vi "insert into cost so far.vi"(9 "new cost":dbl, 10 "Node":cluster{"Weight":dbl, "Row":dbl, "Col":dbl}, 11 "Cost_so_far":T1(array[cluster])) -> (3 "cost_so_far output":T1(array[cluster]))   [LabVIEW 2014]
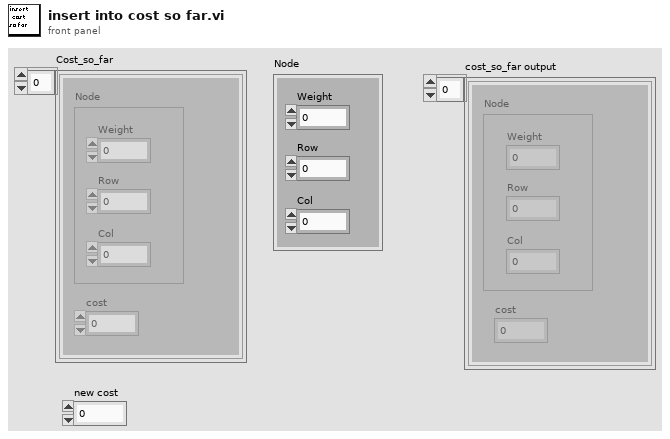
[diagram p1: front panel]
types:
  T1 = cluster{"Node":cluster{"Weight":dbl, "Row":dbl, "Col":dbl}, "cost":dbl}[]
  T2 = cluster{"Node":cluster{"Weight":dbl, "Row":dbl, "Col":dbl}, "cost":dbl}
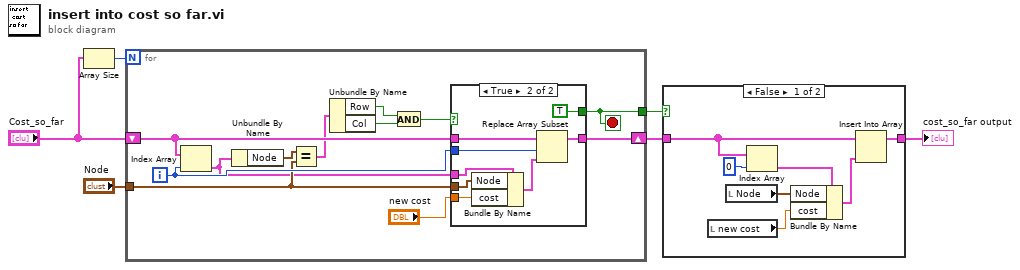
[diagram p0: block diagram]
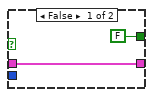
[diagram p3: hidden frame]
diagram:
  n1 = Array Size(array="Cost_so_far") -> (size(s)=w6:i32)
  n2 = for {
    N: w6 -> [_]
    tunnel: "Node" -> [w15]
    shift-right: [w12] -> w2
    shift-left: "Cost_so_far" -> [w17]
    tunnel: [w11] -> w3
    i -> [w16]
    stop <- w11 stop-if-true
    n3 = Index Array(array=w17, index=w16) -> (element=w14:T2)
    n4 = Unbundle By Name(w14) -> ("Node"=w18:cluster{"Weight":dbl, "Row":dbl, "Col":dbl})
    n5 = Equal?(x=w18, y=w15) -> (x = y?=w9:cluster{"Weight":bool, "Row":bool, "Col":bool})
    n6 = Unbundle By Name(w9) -> ("Row"=w8:bool, "Col"=w7:bool)
    n7 = And(x=w8, y=w7) -> (x .and. y?=w10:bool)
    n8 = case shown="True" w10 {
      tunnel: w17 -> [w20 w24]
      tunnel: w16 -> [_ w28]
      tunnel: w15 -> [_ w26]
      tunnel: w14 -> [_ w27]
      tunnel: "new cost" -> [_ w25]
      tunnel: [w20 w22] -> w12
      tunnel: [FALSE TRUE] -> w11
      frame False {
      }
      frame True {
        n9 = Bundle By Name(cluster=w27, "Node"=w26, "cost"=w25) -> (w23:T2)
        n10 = Replace Array Subset(array=w24, new element=w23, index=w28) -> (w22:T1)
      }
    }
  }
  n11 = case shown="False" w3 {
    tunnel: w2 -> [w34 w36]
    tunnel: [w29 w36] -> w1
    frame False {
      n12 = local read "new cost"() -> (w32:dbl)
      n13 = local read "Node"() -> (w31:cluster{"Weight":dbl, "Row":dbl, "Col":dbl})
      n14 = Index Array(array=w34, index=0) -> (element=w33:T2)
      n15 = Bundle By Name(cluster=w33, "Node"=w31, "cost"=w32) -> (w30:T2)
      n16 = Insert Into Array(array=w34, new element=w30) -> (w29:T1)  [unwired: 1 in]
    }
    frame True {
    }
  }
  "cost_so_far output" <- w1
